vi "CirclePlot.vi"() -> ()   [LabVIEW 2019]
panel:
  in  "Reset":bool
  in  "Color":u32(colorbox)
  in  "Stop":bool
  in  "X-Center":dbl(slide) scale=-10.0..10.0
  in  "Y-Center":dbl(slide) scale=-10.0..10.0
  in  "Radius":dbl(slide) scale=0.0..10.0
  out "XY Graph":cluster{dbl[], dbl[]}(graph)
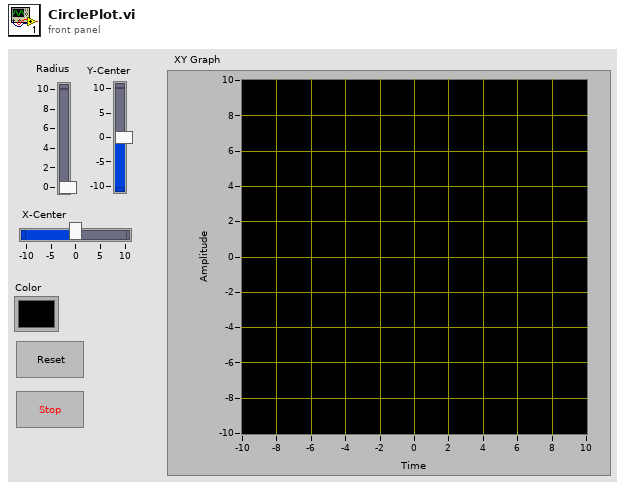
[diagram p1: front panel]
types:
  T1 = cluster{"radius":dbl, "Y-center":dbl, "x-center":dbl, u32}
  T2 = cluster{"Radius":dbl, "Y-Center":dbl, "X-Center":dbl, "Color":u32}
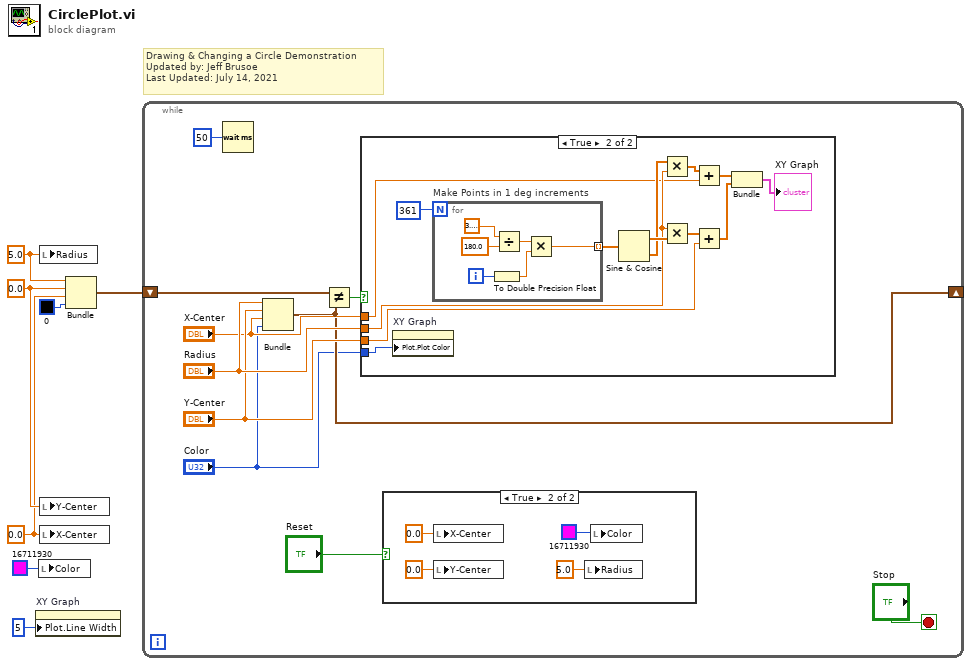
[diagram p0: block diagram]
diagram:
  w6 = 5.0 ("radius")
  w5 = 0.0 ("Y-center")
  w4 = 0.0 ("x-center")
  # "Drawing & Changing a Circle Demonstration\nUpdated by: Jeff Brusoe\nLast Updated: July 14, 2021"
  n1 = property on="XY Graph" class="XYGraph (strict)"("Plot.Line Width"=u8 5) -> ()  [unwired: 2 in, 2 out]
  n2 = local write "Color"(u32 16711930 ("Color")) -> ()
  n3 = local write "Radius"(w6) -> ()
  n4 = local write "Y-Center"(w5) -> ()
  n5 = local write "X-Center"(w4) -> ()
  n6 = Bundle("radius"=w6, "Y-center"=w5, "x-center"=w4, u32 0) -> (w7:T1)  [unwired: 1 in]
  n7 = while {
    shift-right: [w11] -> _
    shift-left: w7 -> [w12]
    stop <- "Stop" stop-if-true
    n8 = Wait (ms)(milliseconds to wait=u32 50) -> ()  [unwired: 1 out]
    n9 = Bundle("Radius"="Radius", "Y-Center"="Y-Center", "X-Center"="X-Center", "Color"="Color") -> (w11:T2)  [unwired: 1 in]
    n10 = Not Equal?(x=w12, y=w11) -> (x != y?=w13:bool)
    n11 = case shown="True" w13 {
      tunnel: "Radius" -> [_ w25]
      tunnel: "Y-Center" -> [_ w24]
      tunnel: "X-Center" -> [_ w23]
      tunnel: "Color" -> [_ w22]
      frame False {
      }
      frame True {
        n12 = property on="XY Graph" class="XYGraph (strict)"("Plot.Plot Color"=w22) -> ()  [unwired: 2 in, 2 out]
        n13 = for "Make Points in 1 deg increments" {
          N: 361 -> [_]
          tunnel: [w39] -> w33 mode=indexing
          i -> [w40]
          n14 = To Double Precision Float(number=w40) -> (double precision float=w35:dbl)
          n15 = Divide(x=3.141592653589793, y=180.0) -> (x/y=w38:dbl)
          n16 = Multiply(x=w38, y=w35) -> (x*y=w39:dbl)
        }
        n17 = Sine & Cosine(0:w33) -> (1:w32:dbl[], 2:w31:dbl[])
        n18 = Multiply(x=w31, y=w25) -> (x*y=w27:dbl[])
        n19 = Multiply(x=w25, y=w32) -> (x*y=w29:dbl[])
        n20 = Add(x=w27, y=w23) -> (x+y=w26:dbl[])
        n21 = Add(x=w29, y=w24) -> (x+y=w28:dbl[])
        n22 = Bundle(w26, w28) -> (→"XY Graph":cluster{dbl[], dbl[]})  [unwired: 1 in]
      }
    }
    n23 = case shown="True" "Reset" {
      frame False {
      }
      frame True {
        n24 = local write "X-Center"(0.0 ("X-Center")) -> ()
        n25 = local write "Y-Center"(0.0 ("Y-Center")) -> ()
        n26 = local write "Radius"(5.0 ("Radius")) -> ()
        n27 = local write "Color"(u32 16711930 ("Color")) -> ()
      }
    }
  }
